vi "Replace4spaces.vi"(11 "String in":string) -> (2 "number of replacements":i32, 3 "String out":string)   [LabVIEW 2022 SP3]
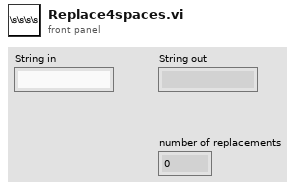
[diagram p1: front panel]
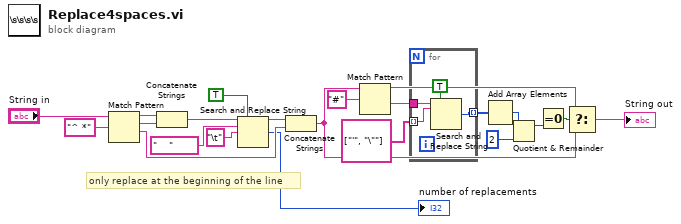
[diagram p0: block diagram]
diagram:
  # "only replace at the beginning of the line"
  n1 = Match Pattern(string="String in", regular expression="^ *" ("format string")) -> (before substring=w16:string, match substring=w17:string, after substring=w22:string)  [unwired: 1 in, 1 out]
  n2 = Concatenate Strings(w16, w17) -> (w18:string)
  n3 = Search and Replace String(replace all?=TRUE ("replace all? (F)"), input string=w18, search string="    " ("search"), replace string="\t" ("replace")) -> (result string=w21:string, number of replacements=→"number of replacements":i32)  [unwired: 4 in, 2 out]
  n4 = Concatenate Strings(w21, w22) -> (w4:string)
  n5 = Match Pattern(string=w4, regular expression="#") -> (before substring=w6:string, after substring=w3:string)  [unwired: 1 in, 2 out]
  n6 = for {
    tunnel: [w25] -> w10 mode=indexing
    tunnel: w3 -> [w24]
    tunnel: string[] ["'", "\""] -> [w23] mode=indexing
    n7 = Search and Replace String(replace all?=TRUE ("replace all? (F)"), input string=w24, search string=w23) -> (number of replacements=w25:i32)  [unwired: 5 in, 3 out]
  }
  n8 = Add Array Elements(numeric array=w10) -> (sum=w1:i32)
  n9 = Quotient & Remainder(x=w1, y=2) -> (x-y*floor(x/y)=w8:i32)  [unwired: 1 out]
  n10 = Equal To 0?(x=w8) -> (x = 0?=w7:bool)
  n11 = Select(t=w6, s=w7, f=w4) -> (s? t:f=→"String out":string)
